vi "Main.vi"(11 "error in (no error)":errorcluster) -> (15 "error out":errorcluster)   [LabVIEW 2014, in "Coding Platform.lvlib"]
uses:
  Coding Platform.lvlib
  Typedefs/Queue Driver Operations.ctl
  Typedefs/DataCluster.ctl
  Typedefs/Test Info.ctl
  Typedefs/Status Of Test.ctl
  Typedefs/Candidate.ctl
  Typedefs/Candidate State.ctl
  Typedefs/Answer Info.ctl
  Typedefs/Answer State.ctl
  Typedefs/User Event Operations.ctl
  Typedefs/TestQuestions.ctl
  APIs/Datatypes/Login.ctl
  APIs/Datatypes/Get Test Info.ctl
  APIs/Datatypes/Test Description.ctl
  APIs/Datatypes/Get Question.ctl
  APIs/Datatypes/Question Response.ctl
  APIs/Datatypes/Candidate Test Info Query.ctl
  APIs/Datatypes/Candidate Test Info.ctl
  APIs/Datatypes/Start Test.ctl
panel:
  in  "Tree":string(tree)
  in  "Test Name":string
  in  "Start Test":bool
  in  "Candidates":i32[](listbox)
  in  "Questions":i32[](listbox)
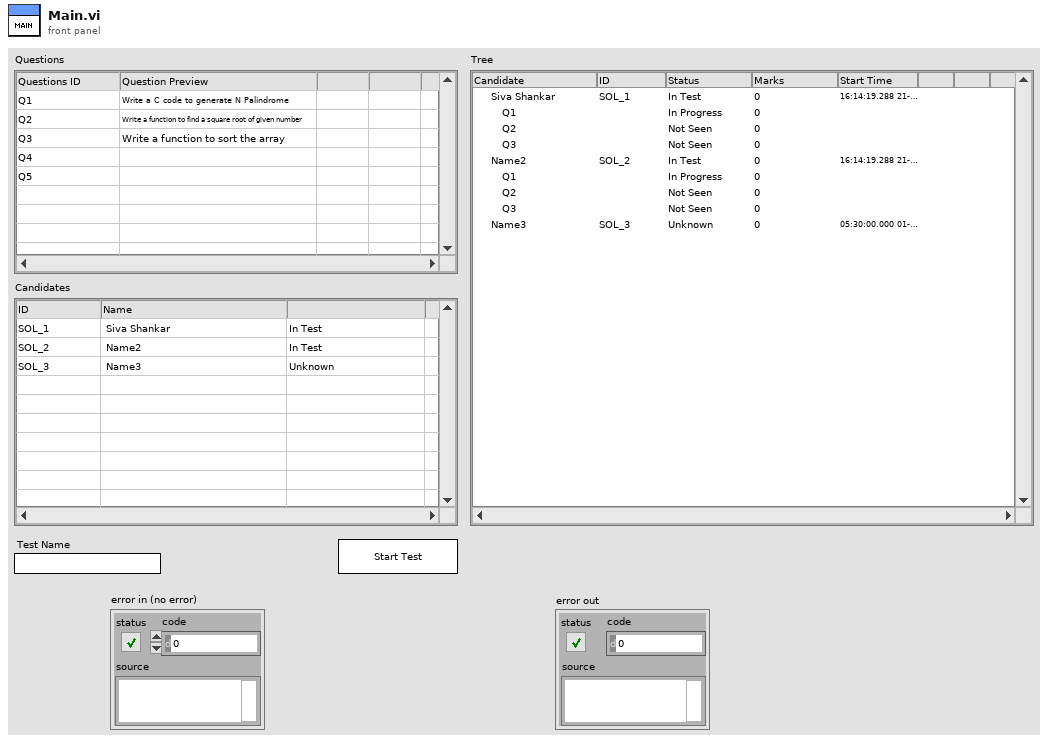
[diagram p1: front panel]
types:
  T1 = typedef "Coding Platform.lvlib/DataCluster.ctl" = cluster{"QuestionID[]":string[], "QuestionsInfo":variant, "Programming Round":T2, "Candidates":T4[]}
  T2 = typedef "Coding Platform.lvlib/Test Info.ctl" = cluster{"Test Name":string, "QuestionsID[]":string[], "CandidatesID[]":string[], "Status":T3}
  T3 = typedef "Coding Platform.lvlib/Status Of Test.ctl" = enum16{"Yet to Start", "In Progress", "Completed"}
  T4 = typedef "Coding Platform.lvlib/Candidate.ctl" = cluster{"ID":string, "Name":string, "Email":string, "Start Time":timestamp, "State":T5, "Answer[]":T6[], "ActiveQuestionID":string}
  T5 = typedef "Coding Platform.lvlib/Candidate State.ctl" = enum16{"Unknown", "LoggedIn", "In Test", "Completed Test"}
  T6 = typedef "Coding Platform.lvlib/Answer Info.ctl" = cluster{"QuestionID":string, "State":T7, "Score":u64}
  T7 = typedef "Coding Platform.lvlib/Answer State.ctl" = enum16{"Not Seen", "In Progress", "Completed"}
  T8 = typedef "Coding Platform.lvlib/Queue Driver Operations.ctl" = enum16{"Create", "Enqueue", "Dequeue", "Destory"}
  T9 = typedef "Coding Platform.lvlib/User Event Operations.ctl" = enum16{"Create", "Genereate", "Destroy", "Get Reference"}
  T10 = typedef "Coding Platform.lvlib/TestQuestions.ctl" = cluster{"Question":string, "TestCase Folder":path}
  T11 = enum16{"open", "replace", "create", "open or create", "replace or create", "replace or create with confirmation"}
  T12 = typedef "Coding Platform.lvlib/Login.ctl" = cluster{"Candidate_ID":string, "Password":string, "notifier":refnum<notifier>}
  T13 = typedef "Coding Platform.lvlib/Test Description.ctl" = cluster{"TestName":string, "Description":string, "Status":string, "cID":string[], "qID":string[]}
  T14 = typedef "Coding Platform.lvlib/Get Test Info.ctl" = cluster{"Candidate_ID":string, "notifier":refnum<notifier>}
  T15 = typedef "Coding Platform.lvlib/Question Response.ctl" = cluster{"QuestionTitle":string, "Question":string, "Description":string}
  T16 = typedef "Coding Platform.lvlib/Get Question.ctl" = cluster{"CandidateID":string, "Question_ID":string, "notifier":refnum<notifier>}
  T17 = typedef "Coding Platform.lvlib/Candidate Test Info.ctl" = cluster{"TestName":string, "Description":string, "State":string, "CurrentQID":string, "QIDs":string[], "QStates":string[], "QScores":u64[]}
  T18 = typedef "Coding Platform.lvlib/Candidate Test Info Query.ctl" = cluster{"Candidate_ID":string, "notifier":refnum<notifier>}
  T19 = typedef "Coding Platform.lvlib/Start Test.ctl" = cluster{"Candidate_ID":string, "notifier":refnum<notifier>}
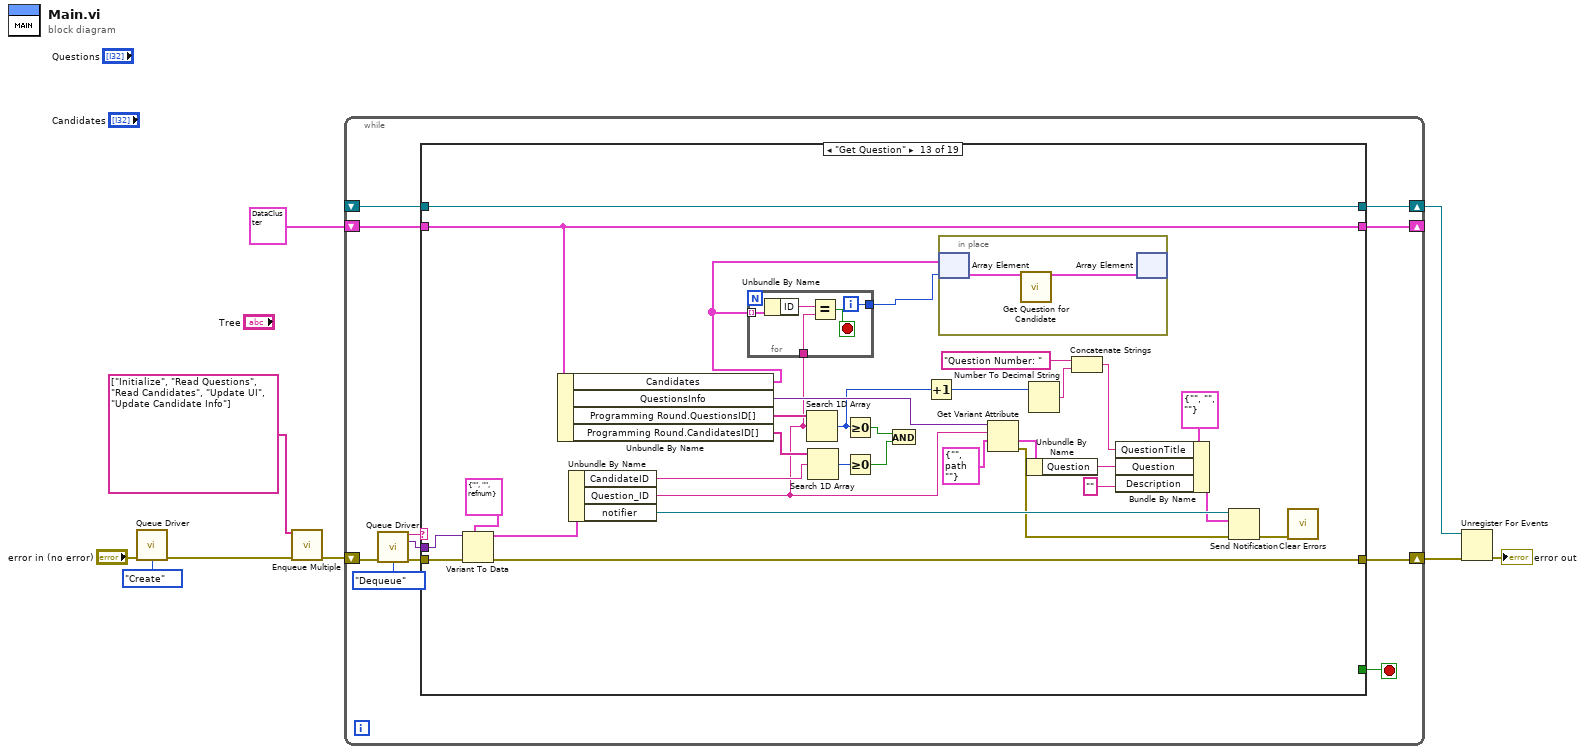
[diagram p0: block diagram]
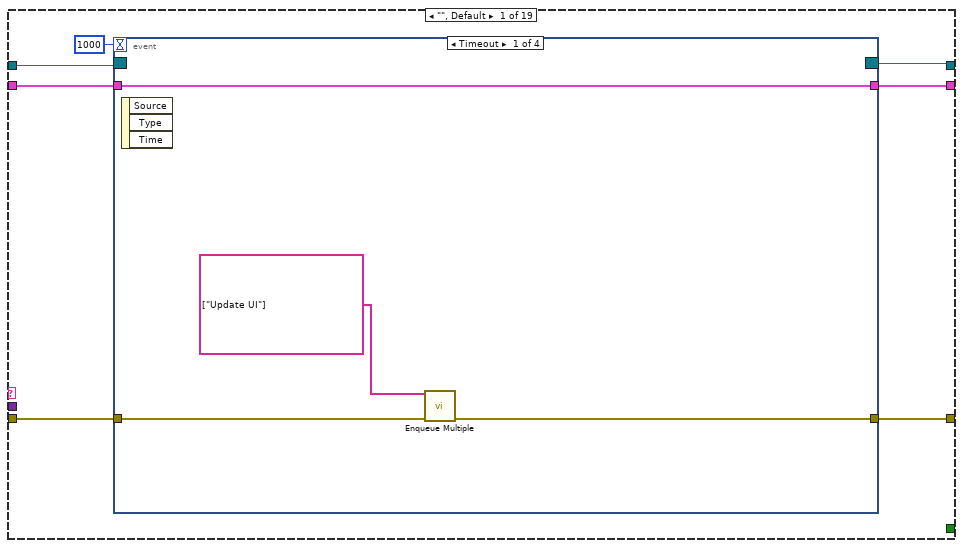
[diagram p2: hidden frame]
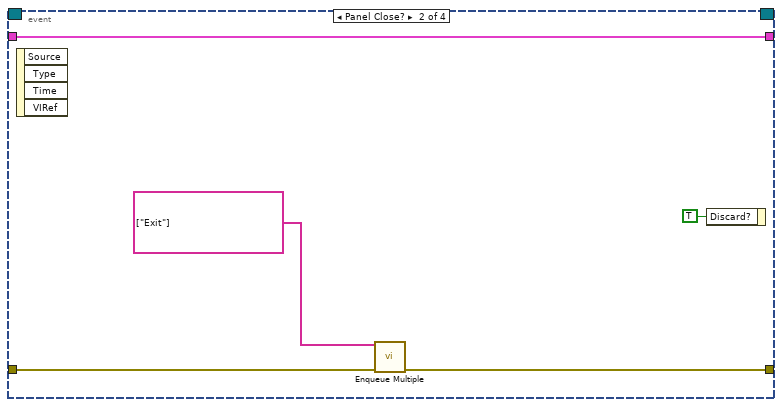
[diagram p3: hidden frame]
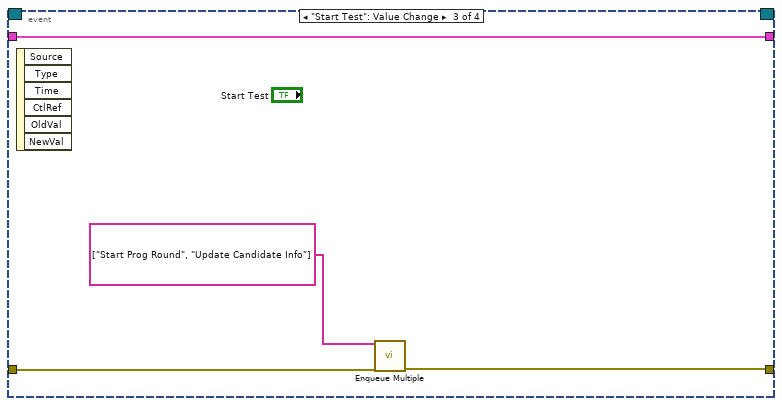
[diagram p4: hidden frame]
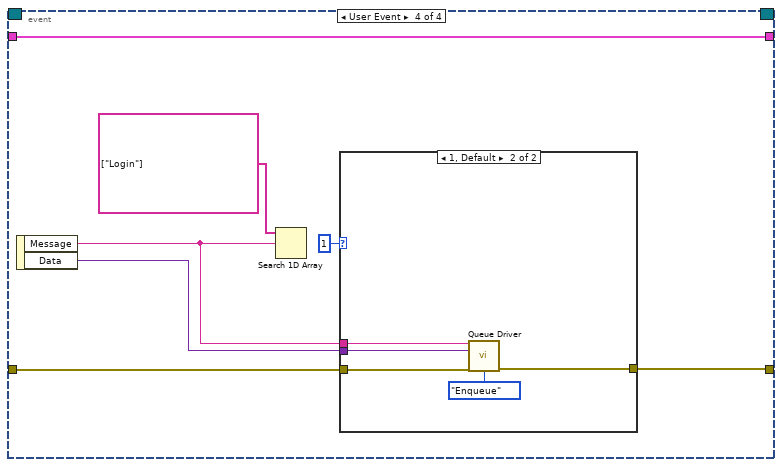
[diagram p5: hidden frame]
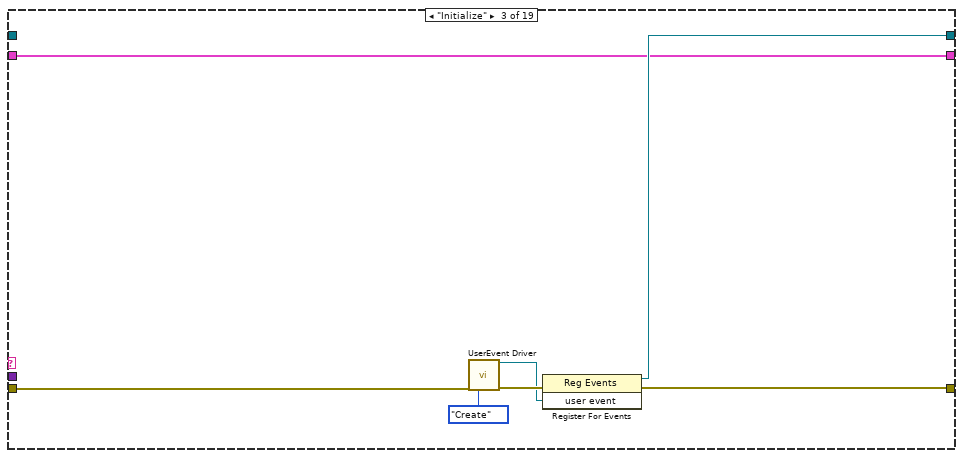
[diagram p8: hidden frame]
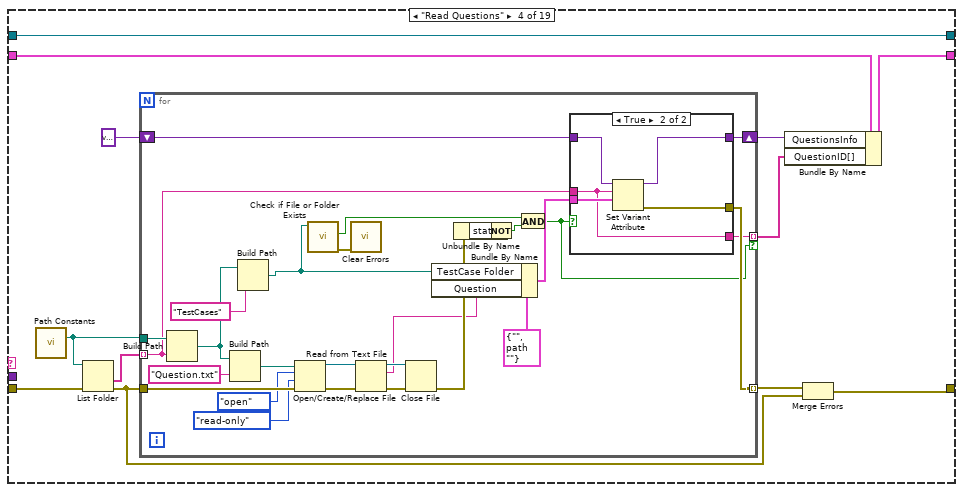
[diagram p9: hidden frame]
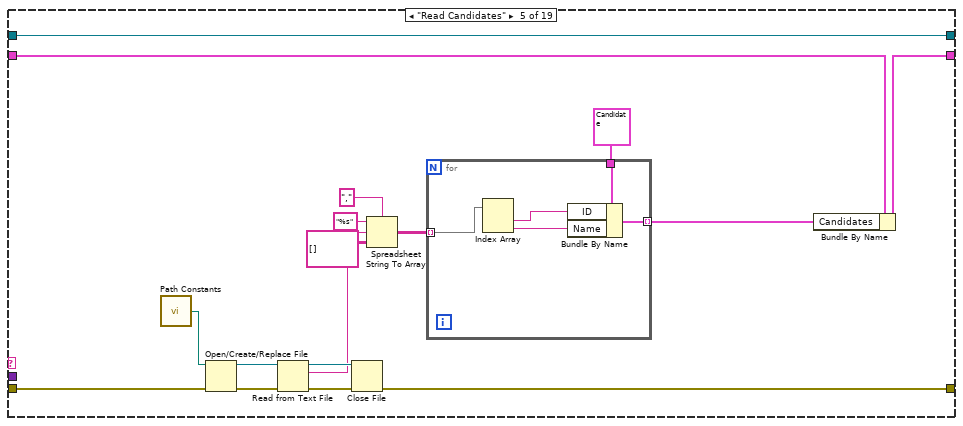
[diagram p11: hidden frame]
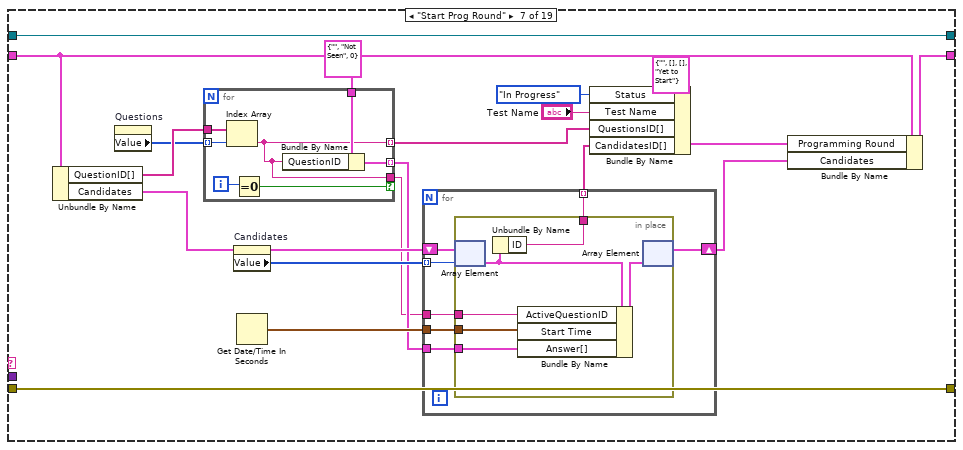
[diagram p13: hidden frame]
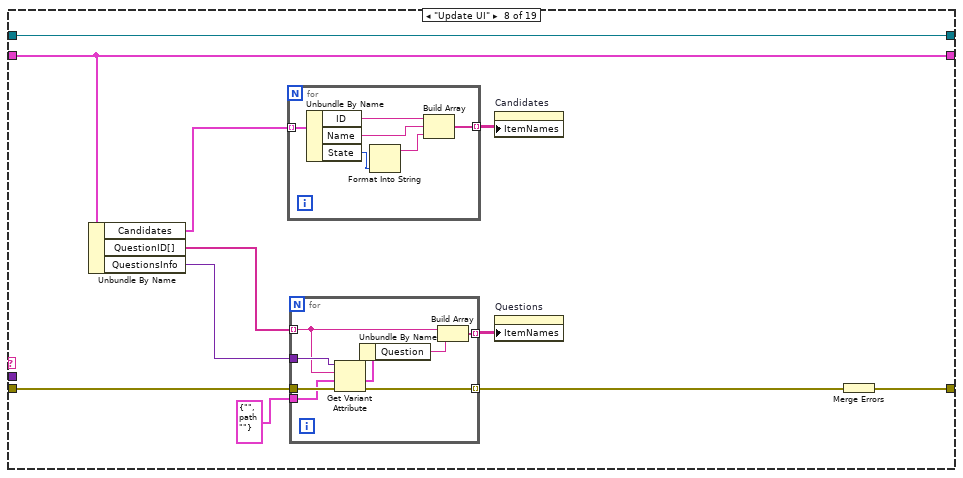
[diagram p14: hidden frame]
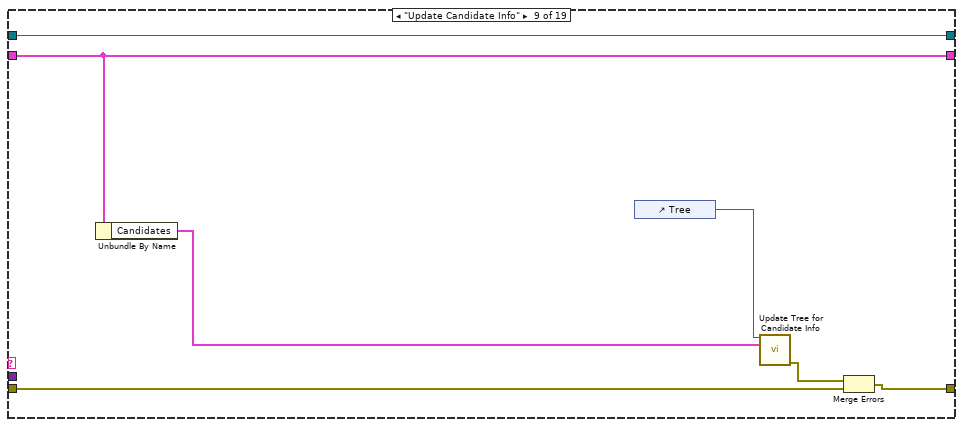
[diagram p15: hidden frame]
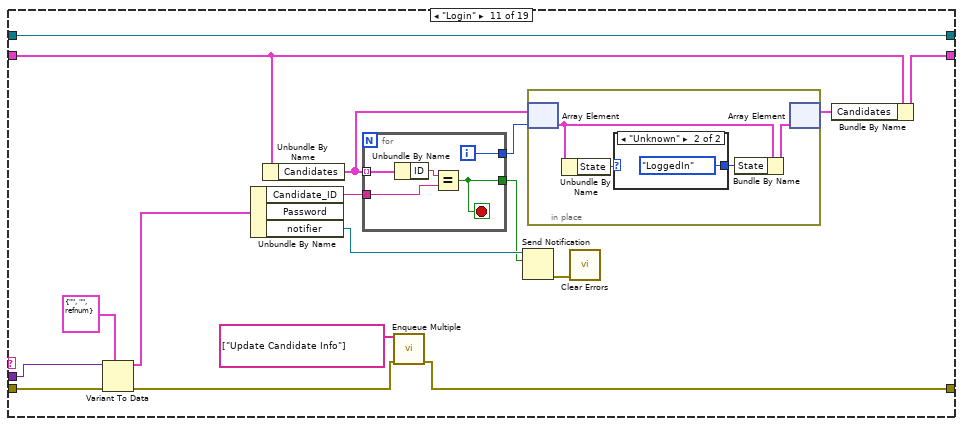
[diagram p17: hidden frame]
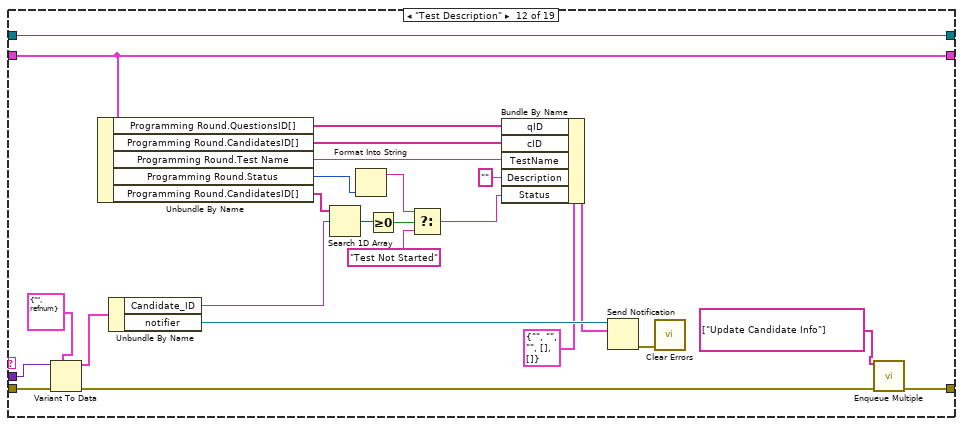
[diagram p19: hidden frame]
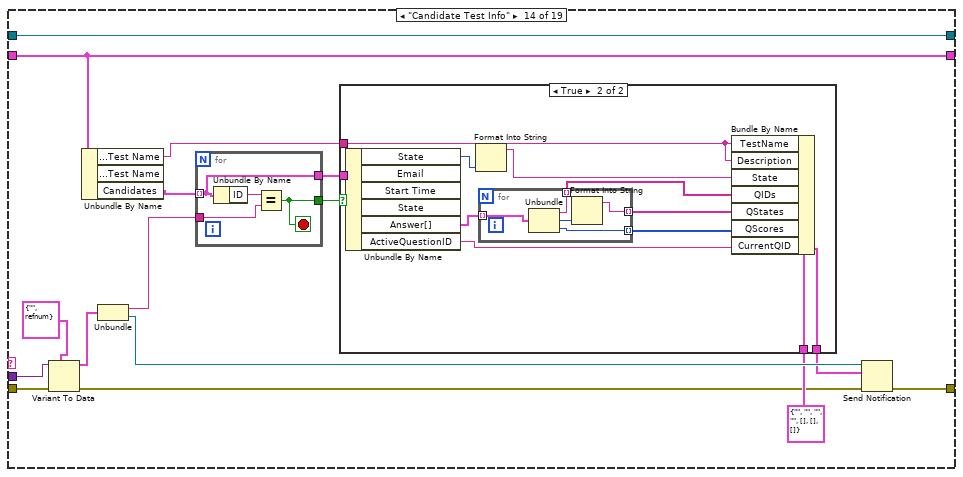
[diagram p20: hidden frame]
diagram:
  n1 = call "Queue Driver.vi"("error in (no error)"="error in (no error)", "Operation"=Queue_Driver_Operations."Create") -> ("error out"=w8:errorcluster)  [unwired: 11 in, 2 out]
  n2 = call "Enqueue Multiple.vi"("State"=string[] ["Initialize", "Read Questions", "Read Candidates", "Update UI", "Update Candidate Info"], "error in (no error)"=w8) -> ("error out"=w6:errorcluster)  [unwired: 13 in]
  n3 = while {
    shift-right: [w20] -> w3
    shift-left: w6 -> [w19]
    shift-right: [w15] -> w4
    shift-left: _ -> [w14]
    shift-right: [w13] -> _
    shift-left: T1 {"QuestionID[]"=[], "QuestionsInfo"=variant, "Programming Round"={"Test Name"="", "QuestionsID[]"=[], "CandidatesID[]"=[], "Status"=enum."Yet to Start"}, "Candidates"=[]} -> [w12]
    stop <- w11 stop-if-true
    n4 = call "Queue Driver.vi"("error in (no error)"=w19, "Operation"=Queue_Driver_Operations."Dequeue") -> ("State Out"=w16:string, "Data Out"=w10:variant, "error out"=w18:errorcluster)  [unwired: 11 in]
    n5 = case shown="\"Get Question\"" w16 {
      tunnel: [w25 w56 w60 w71 w118 w133 w152 w173 w201 w207 w209 w236 w289 w306 w338 w355 w359 w363 w371] -> w20
      tunnel: w18 -> [w24 w56 w62 w73 w125 w133 w152 w177 w198 w207 w224 w260 w291 w313 w353 w356 w359 w365 w371]
      tunnel: [w22 w55 w58 w75 w124 w132 w151 w183 w204 w206 w223 w259 w290 w314 w352 w358 w361 w367 w370] -> w15
      tunnel: w14 -> [w26 w55 _ w75 w124 w132 w151 w183 w204 w206 w223 w259 w290 w314 w352 w358 w361 w367 w370]
      tunnel: [w23 w54 w57 w67 w122 w131 w142 w182 w203 w205 w214 w256 w285 w309 w344 w357 w360 w366 w369] -> w13
      tunnel: w12 -> [w27 w54 w57 w74 w123 w131 w150 w182 w203 w205 w219 w256 w285 w309 w345 w357 w360 w366 w369]
      tunnel: [_ _ _ _ _ _ _ _ _ _ _ _ _ _ _ _ _ _ TRUE] -> w11
      tunnel: w10 -> [_ _ _ _ _ _ _ _ _ _ w222 w258 w288 w312 w350 _ _ _ _]
      frame "", Default {
        n6 = event shown="[0] Timeout" {
          selector: w26 -> [_ _ _ _]
          dyn-events: [_ _ _ _] -> w22
          timeout: 1000 -> [_ _ _ _]
          tunnel: w27 -> [w31 w32 w40 w47]
          tunnel: [w29 w34 w38 w45] -> w25
          tunnel: w24 -> [w30 w36 w39 w46]
          tunnel: [w31 w32 w40 w47] -> w23
          event Timeout {
            n7 = event-data() -> ()  [unwired: 1 in, 3 out]
            n8 = call "Enqueue Multiple.vi"("State"=string[] ["Update UI"], "error in (no error)"=w30) -> ("error out"=w29:errorcluster)  [unwired: 13 in]
          }
          event Panel Close? {
            n9 = event-data() -> ()  [unwired: 1 in, 4 out]
            n10 = call "Enqueue Multiple.vi"("State"=string[] ["Exit"], "error in (no error)"=w36) -> ("error out"=w34:errorcluster)  [unwired: 13 in]
            n11 = event-data("Discard?"=TRUE) -> ()  [unwired: 1 in, 1 out]
          }
          event "Start Test": Value Change {
            n12 = event-data() -> ()  [unwired: 1 in, 6 out]
            n13 = call "Enqueue Multiple.vi"("State"=string[] ["Start Prog Round", "Update Candidate Info"], "error in (no error)"=w39) -> ("error out"=w38:errorcluster)  [unwired: 13 in]
          }
          event User Event {
            n14 = event-data() -> ("Message"=w43:string, "Data"=w44:variant)  [unwired: 1 in]
            n15 = Search 1D Array(1D array=string[] ["Login"], element=w43) -> ()  [unwired: 1 in, 1 out]
            n16 = case shown="1, Default" 1 ("index of element") {
              tunnel: w46 -> [w48 w53]
              tunnel: [w48 w52] -> w45
              tunnel: w44 -> [_ w50]
              tunnel: w43 -> [_ w49]
              frame -1 {
              }
              frame 1, Default {
                n17 = call "Queue Driver.vi"("State"=w49, "Data"=w50, "error in (no error)"=w53, "Operation"=Queue_Driver_Operations."Enqueue") -> ("error out"=w52:errorcluster)  [unwired: 9 in, 2 out]
              }
            }
          }
        }
      }
      frame "-------------Initializations----------------" {
      }
      frame "Initialize" {
        n18 = call "UserEvent Driver.vi"("error in (no error)"=w62, "Operations(Get Reference)"=User_Event_Operations."Create") -> ("user event"=w59:refnum<user-event>, "error out"=w61:errorcluster)  [unwired: 12 in]
        n19 = register-events(error in=w61, w59) -> (reference out=w58:refnum<event-registration>, error out=w60:errorcluster)  [unwired: 1 in]
      }
      frame "Read Questions" {
        n20 = call "Path Constants.vi"() -> ("QuestionBank Drive"=w64:path)  [unwired: 13 in, 2 out]
        n21 = List Folder(path=w64, error in=w73) -> (folder names=w70:string[], error out=w68:errorcluster)  [unwired: 2 in, 2 out]
        n22 = for {
          tunnel: [w87] -> w72 mode=indexing
          tunnel: w68 -> [w102]
          tunnel: w64 -> [w101]
          tunnel: w70 -> [w79] mode=indexing
          shift-right: [w88] -> w66
          shift-left: variant -> [w100]
          tunnel: [w78] -> w65 mode=indexing if=w77
          n23 = Build Path(base path=w101, name or relative path=w79) -> (appended path=w99:path)
          n24 = Build Path(base path=w99, name or relative path="Question.txt") -> (appended path=w95:path)
          n25 = Build Path(base path=w99, name or relative path="TestCases") -> (appended path=w82:path)
          n26 = Open/Create/Replace File(file path (use dialog)=w95, error in=w102, operation (0:open)=T11."open", access (0:read/write)=enum16{"read/write", "read-only", "write-only"}."read-only") -> (refnum out=w91:refnum<file>, error out=w96:errorcluster)  [unwired: 2 in, 1 out]
          n27 = call <vilib>:"Check if File or Folder Exists.vi"("path"=w82) -> ("error out"=w83:errorcluster, "file or folder exists?"=w81:bool)  [unwired: 8 in, 1 out]
          n28 = call <vilib>:"Clear Errors.vi"("error in (no error)"=w83) -> ()  [unwired: 5 in, 2 out]
          n29 = Read from Text File(file (use dialog)=w91, error in=w96) -> (refnum out=w90:refnum<file>, text=w85:string, error out=w92:errorcluster)  [unwired: 2 in, 1 out]
          n30 = Close File(refnum=w90, error in=w92) -> (error out=w89:errorcluster)  [unwired: 1 out]
          n31 = Bundle By Name(cluster=T10 {"Question"="", "TestCase Folder"=path ""} ("TestQuestions"), "TestCase Folder"=w82, "Question"=w85) -> (w80:T10)
          n32 = Unbundle By Name(w89) -> ("status"=w84:bool)
          n33 = Not(x=w84) -> (.not. x?=w76:bool)
          n34 = And(x=w81, y=w76) -> (x .and. y?=w77:bool)
          n35 = case shown="True" w77 {
            tunnel: w100 -> [w103 w108]
            tunnel: [w103 w107] -> w88
            tunnel: [_ w106] -> w87
            tunnel: w80 -> [_ w105]
            tunnel: w79 -> [_ w104]
            tunnel: [_ w104] -> w78
            frame False {
            }
            frame True {
              n36 = Set Variant Attribute(Variant=w108, name=w104, value=w105) -> (Variant out=w107:variant, error out=w106:errorcluster)  [unwired: 1 in, 1 out]
            }
          }
        }
        n37 = Bundle By Name(cluster=w74, "QuestionsInfo"=w66, "QuestionID[]"=w65) -> (w67:T1)
        n38 = Merge Errors(w72, w68) -> (w71:errorcluster)
      }
      frame "Read Candidates" {
        n39 = call "Path Constants.vi"() -> ("Candidates File"=w120:path)  [unwired: 13 in, 2 out]
        n40 = Open/Create/Replace File(file path (use dialog)=w120, error in=w125) -> (refnum out=w117:refnum<file>, error out=w121:errorcluster)  [unwired: 4 in, 1 out]
        n41 = Read from Text File(file (use dialog)=w117, error in=w121) -> (refnum out=w116:refnum<file>, text=w115:string, error out=w119:errorcluster)  [unwired: 2 in, 1 out]
        n42 = Close File(refnum=w116, error in=w119) -> (error out=w118:errorcluster)  [unwired: 1 out]
        n43 = Spreadsheet String To Array(delimiter (Tab)="," ("format string"), format string="%s", spreadsheet string=w115, array type (2D Dbl)=string[][] []) -> (array=w111:string[][])
        n44 = for {
          tunnel: w111 -> [w128] mode=indexing
          tunnel: [w129] -> w110 mode=indexing
          tunnel: T4 {"ID"="", "Name"="", "Email"="", "Start Time"=timestamp(0 s since 1904-01-01), "State"=enum."Unknown", "Answer[]"=[], "ActiveQuestionID"=""} ("Candidate") -> [w130]
          n45 = Index Array(array=w128) -> (element #1=w127:string, element #2=w126:string)  [unwired: 2 in]
          n46 = Bundle By Name(cluster=w130, "ID"=w127, "Name"=w126) -> (w129:T4)
        }
        n47 = Bundle By Name(cluster=w123, "Candidates"=w110) -> (w122:T1)
      }
      frame "--- --------------Operations-------------------" {
      }
      frame "Start Prog Round" {
        n48 = Unbundle By Name(w150) -> ("QuestionID[]"=w149:string[], "Candidates"=w147:T4[])
        n49 = property on="Questions" class="MCListbox (strict)"() -> ("Value"=w148:i32[])  [unwired: 2 in, 2 out]
        n50 = for {
          tunnel: w149 -> [w172]
          tunnel: w148 -> [w171] mode=indexing
          tunnel: [w167] -> w137 mode=indexing
          tunnel: T6 {"QuestionID"="", "State"=enum."Not Seen", "Score"=0} ("Answer") -> [w170]
          tunnel: [w169] -> w143 mode=indexing
          tunnel: [w167] -> w134 if=w166
          i -> [w168]
          n51 = Index Array(array=w172, index=w171) -> (element=w167:string)
          n52 = Equal To 0?(x=w168) -> (x = 0?=w166:bool)
          n53 = Bundle By Name(cluster=w170, "QuestionID"=w167) -> (w169:T6)
        }
        n54 = property on="Candidates" class="MCListbox (strict)"() -> ("Value"=w146:i32[])  [unwired: 2 in, 2 out]
        n55 = Get Date/Time In Seconds() -> (seconds since 1Jan1904=w145:timestamp)
        n56 = for {
          tunnel: w146 -> [w158] mode=indexing
          shift-right: [w157] -> w141
          shift-left: w147 -> [w159]
          tunnel: w145 -> [w156]
          tunnel: w143 -> [w155]
          tunnel: [w154] -> w136 mode=indexing
          tunnel: w134 -> [w153]
          n57 = in-place {
            in-place-border: w156 -> [w164]
            in-place-border: w155 -> [w163]
            in-place-border: [w161] -> w154
            in-place-border: w153 -> [w160]
            n58 = in-place-array #1(w159, w158) -> (w162:T4)
            n59 = Unbundle By Name(w162) -> ("ID"=w161:string)
            n60 = Bundle By Name(cluster=w162, "ActiveQuestionID"=w160, "Start Time"=w164, "Answer[]"=w163) -> (w165:T4)
            n61 = in-place-array #1(w165) -> (w157:T4[])  [unwired: 1 out]
          }
        }
        n62 = Bundle By Name(cluster=T2 {"Test Name"="", "QuestionsID[]"=[], "CandidatesID[]"=[], "Status"=enum."Yet to Start"} ("Programming Round"), "Status"=Status_Of_Test."In Progress", "Test Name"="Test Name", "QuestionsID[]"=w137, "CandidatesID[]"=w136) -> (w139:T2)
        n63 = Bundle By Name(cluster=w150, "Programming Round"=w139, "Candidates"=w141) -> (w142:T1)
      }
      frame "Update UI" {
        n64 = Unbundle By Name(w182) -> ("Candidates"=w174:T4[], "QuestionID[]"=w180:string[], "QuestionsInfo"=w179:variant)
        n65 = for {
          tunnel: w174 -> [w197] mode=indexing
          tunnel: [w194] -> w181 mode=indexing
          n66 = Unbundle By Name(w197) -> ("ID"=w196:string, "Name"=w195:string, "State"=w193:T5)
          n67 = Format Into String(w193) -> (resulting string=w192:string)  [unwired: 3 in, 1 out]
          n68 = Build Array(w196, w195, w192) -> (w194:string[])
        }
        n69 = for {
          tunnel: w180 -> [w187] mode=indexing
          tunnel: [w191] -> w175 mode=indexing
          tunnel: w179 -> [w188]
          tunnel: [w189] -> w178 mode=indexing
          tunnel: w177 -> [w190]
          tunnel: T10 {"Question"="", "TestCase Folder"=path ""} ("TestQuestions") -> [w186]
          n70 = Get Variant Attribute(Variant=w188, name=w187, default value (empty Variant)=w186, error in=w190) -> (value=w185:T10, error out=w189:errorcluster)  [unwired: 2 out]
          n71 = Unbundle By Name(w185) -> ("Question"=w184:string)
          n72 = Build Array(w187, w184) -> (w191:string[])
        }
        n73 = property on="Candidates" class="MCListbox (strict)"("ItemNames"=w181) -> ()  [unwired: 2 in, 2 out]
        n74 = property on="Questions" class="MCListbox (strict)"("ItemNames"=w175) -> ()  [unwired: 2 in, 2 out]
        n75 = Merge Errors(w178) -> (w173:errorcluster)
      }
      frame "Update Candidate Info" {
        n76 = Unbundle By Name(w203) -> ("Candidates"=w202:T4[])
        n77 = control-ref of="Tree"() -> (w199:refnum<vi>)
        n78 = call "Update Tree for Candidate Info.vi"("Tree Ref"=w199, "Candidates"=w202) -> ("error out"=w200:errorcluster)  [unwired: 13 in]
        n79 = Merge Errors(w200, w198) -> (w201:errorcluster)
      }
      frame "-----------------Messages---------------------" {
      }
      frame "Login" {
        n80 = Variant To Data(error in=w224, type=T12 {"Candidate_ID"="", "Password"="", "notifier"=refnum} ("Login"), Variant=w222) -> (data=w220:T12, error out=w210:errorcluster)
        n81 = Unbundle By Name(w220) -> ("Candidate_ID"=w218:string, "notifier"=w217:refnum<notifier>)  [unwired: 1 out]
        n82 = Unbundle By Name(w219) -> ("Candidates"=w215:T4[])
        n83 = for {
          tunnel: w215 -> [w235] mode=indexing
          tunnel: w218 -> [w233]
          tunnel: [w232] -> w216
          tunnel: [w231] -> w212
          i -> [w231]
          stop <- w232 stop-if-true
          n84 = Unbundle By Name(w235) -> ("ID"=w234:string)
          n85 = Equal?(x=w234, y=w233) -> (x = y?=w232:bool)
        }
        n86 = call "Enqueue Multiple.vi"("State"=string[] ["Update Candidate Info"], "error in (no error)"=w210) -> ("error out"=w209:errorcluster)  [unwired: 13 in]
        n87 = Send Notification(notification=w216, notifier=w217) -> (error out=w211:errorcluster)  [unwired: 1 in, 1 out]
        n88 = in-place {
          n89 = in-place-array #2(w215, w212) -> (w226:T4)
          n90 = Unbundle By Name(w226) -> ("State"=w225:T5)
          n91 = case shown="\"Unknown\"" w225 {
            selector: w225 -> [w229 _]
            tunnel: [w229 Candidate_State."LoggedIn" ("State")] -> w227
            frame Default {
            }
            frame "Unknown" {
            }
          }
          n92 = Bundle By Name(cluster=w226, "State"=w227) -> (w228:T4)
          n93 = in-place-array #2(w228) -> (w213:T4[])  [unwired: 1 out]
        }
        n94 = call <vilib>:"Clear Errors.vi"("error in (no error)"=w211) -> ()  [unwired: 5 in, 2 out]
        n95 = Bundle By Name(cluster=w219, "Candidates"=w213) -> (w214:T1)
      }
      frame "Test Description" {
        n96 = Variant To Data(error in=w260, type=T14 {"Candidate_ID"="", "notifier"=refnum} ("Login"), Variant=w258) -> (data=w254:T14, error out=w237:errorcluster)
        n97 = Unbundle By Name(w256) -> ("Programming Round.QuestionsID[]"=w239:string[], "Programming Round.CandidatesID[]"=w240:string[], "Programming Round.Test Name"=w246:string, "Programming Round.Status"=w245:T3, "Programming Round.CandidatesID[]"=w252:string[])
        n98 = Unbundle By Name(w254) -> ("Candidate_ID"=w251:string, "notifier"=w253:refnum<notifier>)
        n99 = Search 1D Array(1D array=w252, element=w251) -> (index of element=w250:i32)  [unwired: 1 in]
        n100 = Format Into String(w245) -> (resulting string=w244:string)  [unwired: 3 in, 1 out]
        n101 = Greater Or Equal To 0?(x=w250) -> (x >= 0?=w249:bool)
        n102 = Select(t=w244, s=w249, f="Test Not Started") -> (s? t:f=w241:string)
        n103 = Bundle By Name(cluster=T13 {"TestName"="", "Description"="", "Status"="", "cID"=[], "qID"=[]} ("notification"), "qID"=w239, "cID"=w240, "TestName"=w246, "Description"="", "Status"=w241) -> (w247:T13)
        n104 = Send Notification(notification=w247, notifier=w253) -> (error out=w255:errorcluster)  [unwired: 1 in, 1 out]
        n105 = call <vilib>:"Clear Errors.vi"("error in (no error)"=w255) -> ()  [unwired: 5 in, 2 out]
        n106 = call "Enqueue Multiple.vi"("State"=string[] ["Update Candidate Info"], "error in (no error)"=w237) -> ("error out"=w236:errorcluster)  [unwired: 13 in]
      }
      frame "Get Question" {
        n107 = Variant To Data(error in=w291, type=T16 {"CandidateID"="", "Question_ID"="", "notifier"=refnum} ("Get Question"), Variant=w288) -> (data=w287:T16, error out=w289:errorcluster)
        n108 = Unbundle By Name(w285) -> ("Candidates"=w262:T4[], "QuestionsInfo"=w278:variant, "Programming Round.QuestionsID[]"=w284:string[], "Programming Round.CandidatesID[]"=w283:string[])
        n109 = Unbundle By Name(w287) -> ("CandidateID"=w282:string, "Question_ID"=w263:string, "notifier"=w275:refnum<notifier>)
        n110 = for {
          tunnel: w262 -> [w298] mode=indexing
          tunnel: w263 -> [w296]
          tunnel: [w294] -> w261
          i -> [w294]
          stop <- w295 stop-if-true
          n111 = Unbundle By Name(w298) -> ("ID"=w297:string)
          n112 = Equal?(x=w297, y=w296) -> (x = y?=w295:bool)
        }
        n113 = Search 1D Array(1D array=w284, element=w263) -> (index of element=w269:i32)  [unwired: 1 in]
        n114 = Search 1D Array(1D array=w283, element=w282) -> (index of element=w281:i32)  [unwired: 1 in]
        n115 = Greater Or Equal To 0?(x=w269) -> (x >= 0?=w280:bool)
        n116 = Greater Or Equal To 0?(x=w281) -> (x >= 0?=w279:bool)
        n117 = And(x=w280, y=w279) -> ()  [unwired: 1 out]
        n118 = Increment(x=w269) -> (x+1=w268:i32)
        n119 = in-place {
          n120 = in-place-array #3(w262, w261) -> (w293:T4)
          n121 = call "Get Question for Candidate.vi"("Candidate"=w293) -> ("element 2"=w292:T4)  [unwired: 13 in, 1 out]
          n122 = in-place-array #3(w292) -> ()  [unwired: 2 out]
        }
        n123 = Get Variant Attribute(Variant=w278, name=w263, default value (empty Variant)=T10 {"Question"="", "TestCase Folder"=path ""} ("TestQuestions")) -> (value=w276:T10, error out=w274:errorcluster)  [unwired: 1 in, 2 out]
        n124 = Unbundle By Name(w276) -> ("Question"=w271:string)
        n125 = Number To Decimal String(number=w268) -> (decimal integer string=w267:string)  [unwired: 1 in]
        n126 = Concatenate Strings("Question Number: ", w267) -> (w265:string)
        n127 = Bundle By Name(cluster=T15 {"QuestionTitle"="", "Question"="", "Description"=""} ("notification"), "QuestionTitle"=w265, "Question"=w271, "Description"="") -> (w272:T15)
        n128 = Send Notification(notification=w272, notifier=w275, error in (no error)=w274) -> (error out=w264:errorcluster)  [unwired: 1 out]
        n129 = call <vilib>:"Clear Errors.vi"("error in (no error)"=w264) -> ()  [unwired: 5 in, 2 out]
      }
      frame "Candidate Test Info" {
        n130 = Variant To Data(error in=w313, type=T18 {"Candidate_ID"="", "notifier"=refnum} ("Login"), Variant=w312) -> (data=w310:T18, error out=w299:errorcluster)
        n131 = Unbundle By Name(w309) -> ("Programming Round.Test Name"=w300:string, "Candidates"=w308:T4[])  [unwired: 1 out]
        n132 = Unbundle(w310) -> ("Candidate_ID"=w307:string, "notifier"=w305:refnum<notifier>)
        n133 = for {
          tunnel: w308 -> [w335] mode=indexing
          tunnel: w307 -> [w336]
          tunnel: [w335] -> w302
          tunnel: [w334] -> w301
          stop <- w334 stop-if-true
          n134 = Unbundle By Name(w335) -> ("ID"=w337:string)
          n135 = Equal?(x=w337, y=w336) -> (x = y?=w334:bool)
        }
        n136 = case shown="True" w301 {
          tunnel: T17 {"TestName"="", "Description"="", "State"="", "CurrentQID"="", "QIDs"=[], "QStates"=[], "QScores"=[]} ("notification") -> [w317 w328]
          tunnel: [w316 w327] -> w303
          tunnel: w302 -> [_ w326]
          tunnel: w300 -> [_ w325]
          frame False {
            n137 = Bundle By Name(cluster=w317, "State"="NO TEST") -> (w316:T17)
          }
          frame True {
            n138 = Unbundle By Name(w326) -> ("State"=w324:T5, "Answer[]"=w322:T6[], "ActiveQuestionID"=w318:string)  [unwired: 3 out]
            n139 = Format Into String(w324) -> (resulting string=w323:string)  [unwired: 3 in, 1 out]
            n140 = for {
              tunnel: w322 -> [w333] mode=indexing
              tunnel: [w331] -> w321 mode=indexing
              tunnel: [w330] -> w320 mode=indexing
              tunnel: [w329] -> w319 mode=indexing
              n141 = Unbundle(w333) -> ("QuestionID"=w331:string, "State"=w332:T7, "Score"=w329:u64)
              n142 = Format Into String(w332) -> (resulting string=w330:string)  [unwired: 3 in, 1 out]
            }
            n143 = Bundle By Name(cluster=w328, "TestName"=w325, "Description"=w325, "State"=w323, "QIDs"=w321, "QStates"=w320, "QScores"=w319, "CurrentQID"=w318) -> (w327:T17)
          }
        }
        n144 = Send Notification(notification=w303, notifier=w305, error in (no error)=w299) -> (error out=w306:errorcluster)  [unwired: 1 out]
      }
      frame "Start Test" {
        n145 = Variant To Data(error in=w353, type=T19 {"Candidate_ID"="", "notifier"=refnum} ("Login"), Variant=w350) -> (data=w348:T19, error out=w351:errorcluster)
        n146 = Unbundle By Name(w345) -> ("Candidates"=w341:T4[])
        n147 = Unbundle(w348) -> ("Candidate_ID"=w342:string, "notifier"=w347:refnum<notifier>)
        n148 = Send Notification(notification=TRUE, notifier=w347, error in (no error)=w351) -> (error out=w339:errorcluster)  [unwired: 1 out]
        n149 = call "Start Test For Candidate.vi"("Candidate_ID"=w342, "Candidates"=w341) -> ("Candidates out"=w343:T4[])  [unwired: 9 in]
        n150 = Bundle By Name(cluster=w345, "Candidates"=w343) -> (w344:T1)
        n151 = call "Enqueue Multiple.vi"("State"=string[] ["Update Candidate Info"], "error in (no error)"=w339) -> ("error out"=w338:errorcluster)  [unwired: 13 in]
      }
      frame "Stop Application" {
        n152 = call "Enqueue Multiple.vi"("State"=string[] ["Exit"], "error in (no error)"=w356) -> ("error out"=w355:errorcluster)  [unwired: 13 in]
      }
      frame "--------------------Misc-----------------------" {
      }
      frame "Error" {
        n153 = Unbundle By Name(w365) -> ()  [unwired: 3 out]
        n154 = call "Path Constants.vi"() -> ("Error Log Path"=w364:path)  [unwired: 13 in, 2 out]
        n155 = flat-sequence {
          tunnel: w364 -> [_]
          frame #0 {
            # "#TODO"
            # "Log to file"
          }
        }
        n156 = call <vilib>:"Simple Error Handler.vi"("error in (no error)"=w365) -> ("error out"=w362:errorcluster)  [unwired: 4 in, 4 out]
        n157 = call <vilib>:"Clear Errors.vi"("error in (no error)"=w362) -> ("error out"=w363:errorcluster)  [unwired: 5 in, 1 out]
      }
      frame "Exit" {
      }
    }
  }
  n158 = Unregister For Events(event registration refnum=w4, error in=w3) -> (error out=→"error out":errorcluster)
